vi "Run Action_Do.vi"(8 "error in (no error)":errorcluster, 10 "Project Builder in":refnum<class "Project Builder.lvclass">, 11 "Set Version from Git Tag":refnum<class "Set Version from Git Tag.lvclass">) -> (0 "error out":errorcluster, 1 "Success?":bool, 3 "Report":refnum<class "Report Data.lvclass">)   [LabVIEW 2019, in "ProjectBuilder.lvlib" / "Set Version from Git Tag.lvclass"]
doc: "Run the action associated with the 'Project Action'-class.\n\nThis implementation gets the Git tag and sets the build specification version to the tag version."
uses:
  Set Version from Git Tag.lvclass
  Project Action/Project Action.lvclass
  ProjectBuilder.lvlib
  <vilib>/AppBuilder/AB_API_Simple/Build Specification Version.ctl
  <vilib>/AppBuilder/AB_API_Simple/NI_App_Builder_API.lvlib
  Version Data/Version Data.lvclass
  Data/Report Data/Report Data.lvclass
  Project Builder/Project Builder.lvclass
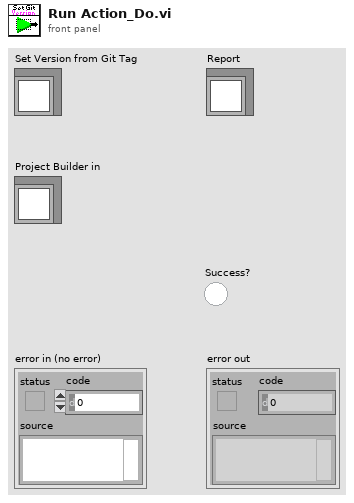
[diagram p1: front panel]
types:
  T1 = typedef "NI_App_Builder_API.lvlib/Build Specification Version.ctl" = cluster{"Major":u16, "Minor":u16, "Fix":u16, "Build":u16}
  T2 = cluster{"Build Specification Version[0]":i32, "Build Specification Version[1]":i32, "Build Specification Version[2]":i32, "Build Specification Version[3]":i32}
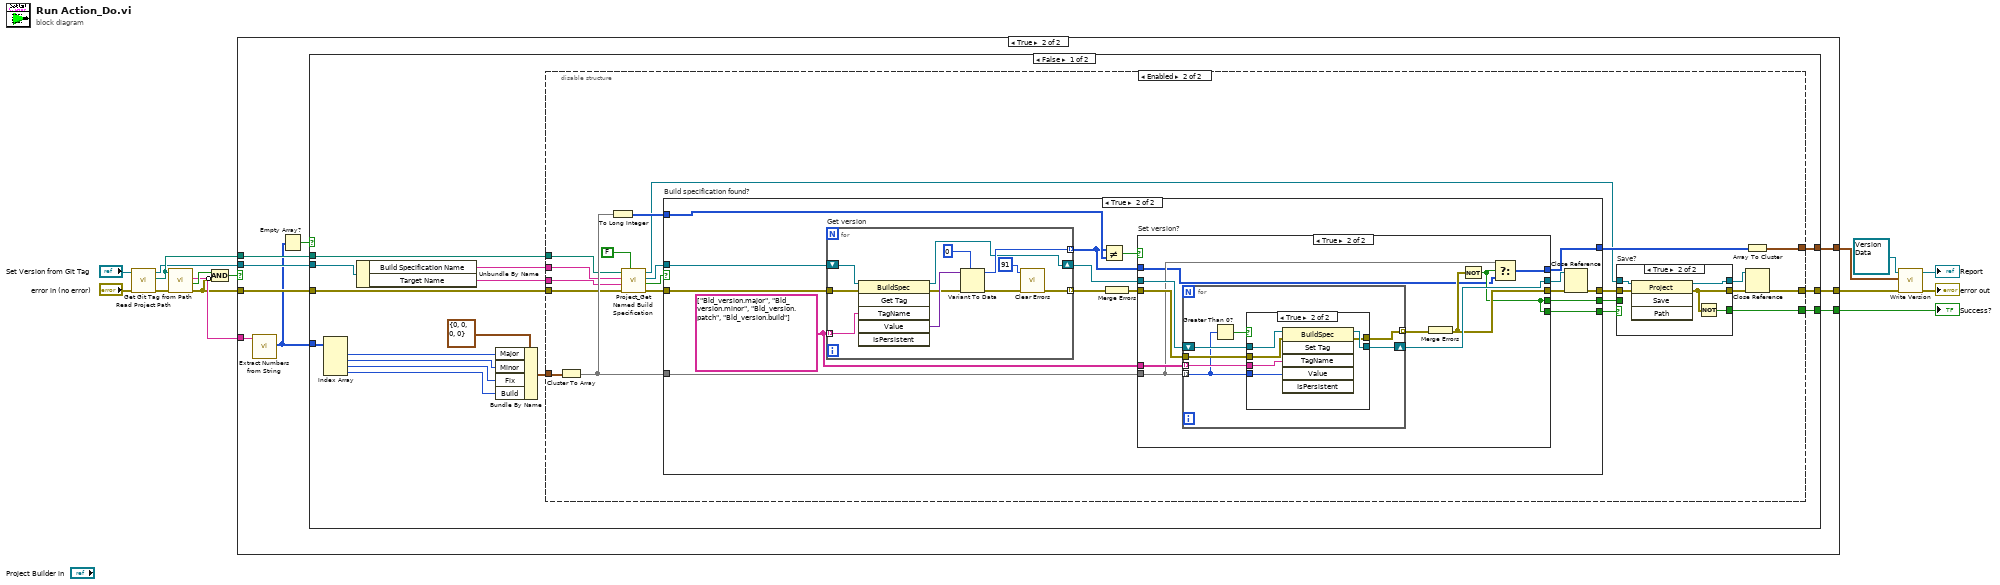
[diagram p0: block diagram]
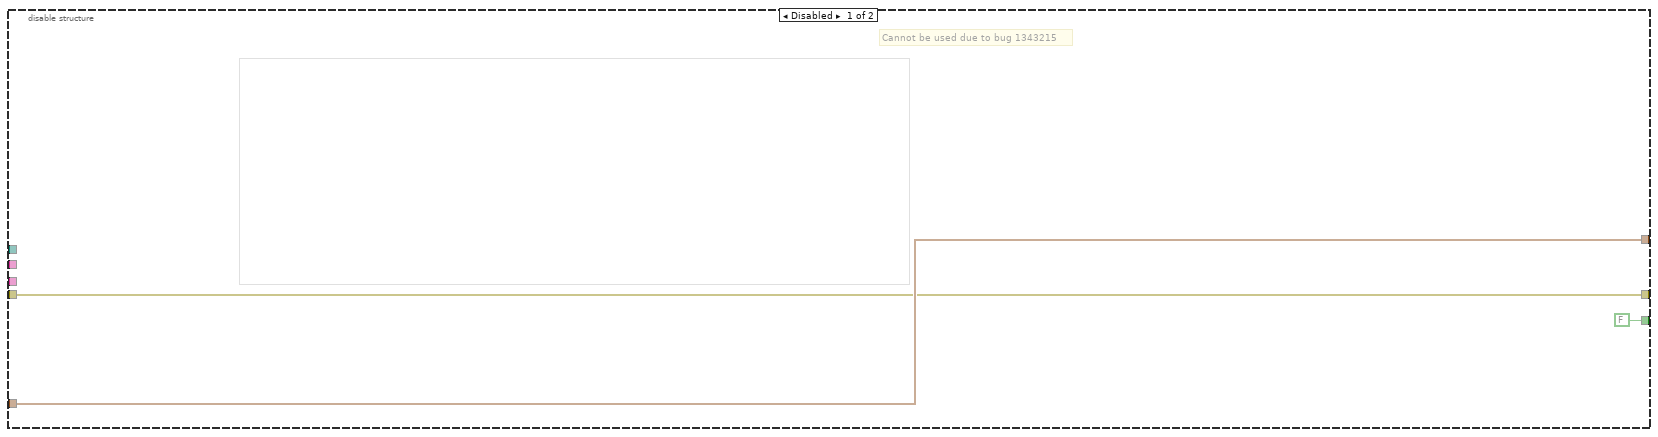
[diagram p3: hidden frame]
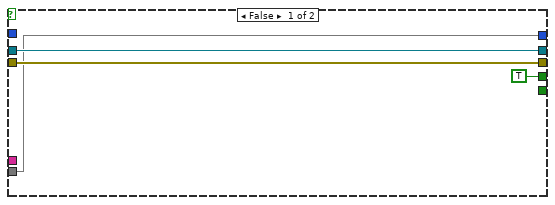
[diagram p5: hidden frame]
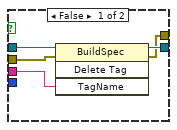
[diagram p6: hidden frame]
diagram:
  n1 = call "Read Project Path.vi"("error in (no error)"="error in (no error)", "Project Action in"="Set Version from Git Tag") -> ("error out"=w13:errorcluster, "Project Path"=w9:path, "Project Action out"=w7:refnum<class "Set Version from Git Tag.lvclass">)  [unwired: 7 in]
  n2 = call "Get Git Tag from Path.vi"("error in (no error)"=w13, "Path"=w9) -> ("error out"=w8:errorcluster, "Success?"=w12:bool, "Tag"=w10:string)  [unwired: 6 in, 1 out]
  n3 = Compound Arithmetic op=AND(w12, invert w8) -> (w11:bool)
  n4 = case shown="True" w11 {
    selector: w11 -> [w16 _]
    tunnel: w10 -> [_ w26]
    tunnel: w9 -> [_ w25]
    tunnel: [w17 w22] -> w6
    tunnel: w8 -> [w17 w23]
    tunnel: [w16 w21] -> w5
    tunnel: w7 -> [_ w24]
    tunnel: [_ w18] -> w1
    frame False {
    }
    frame True {
      n5 = call "Extract Numbers from String.vi"("String"=w26) -> ("Number Array"=w20:i32[])  [unwired: 9 in, 1 out]
      n6 = Empty Array?(array=w20) -> (empty?=w19:bool)
      n7 = case shown="False" w19 {
        tunnel: w25 -> [w28 _]
        tunnel: w24 -> [w36 _]
        tunnel: w23 -> [w29 w134]
        tunnel: [w27 w134] -> w22
        tunnel: [w35 _] -> w21
        tunnel: w20 -> [w34 _]
        tunnel: [w31 _] -> w18
        frame False {
          n8 = Index Array(array=w34) -> (element #1=w40:i32, element #2=w39:i32, element #3=w38:i32, element #4=w37:i32)  [unwired: 4 in]
          n9 = Unbundle By Name(w36) -> ("Build Specification Name"=w33:string, "Target Name"=w30:string)
          n10 = Bundle By Name(cluster=T1 {"Major"=0, "Minor"=0, "Fix"=0, "Build"=0} ("Build Specification Version"), "Major"=w40, "Minor"=w39, "Fix"=w38, "Build"=w37) -> (w32:T1)
          n11 = disable-structure shown="Enabled" {
            disable-tunnel: [FALSE w58] -> w35
            disable-tunnel: w33 -> [_ w53]
            disable-tunnel: w32 -> [w44 w63]
            disable-tunnel: [w44 w55] -> w31
            disable-tunnel: w30 -> [_ w45]
            disable-tunnel: w29 -> [w43 w54]
            disable-tunnel: w28 -> [_ w52]
            disable-tunnel: [w43 w59] -> w27
            frame Disabled {
              # "Cannot be used due to bug 1343215"
            }
            frame Enabled {
              n12 = Cluster To Array(cluster=w63) -> (array=w62:u16[])
              n13 = To Long Integer(number=w62) -> (32bit integer=w61:i32[])
              n14 = call "Project_Get Named Build Specification.vi"("Close project reference(T)"=FALSE, "error in(no error)"=w54, "Target Name(\"\"> My Computer)"=w45, "Build Specification Name"=w53, "Project Path"=w52) -> ("error out"=w48:errorcluster, "Success?"=w50:bool, "Build Spec reference"=w49:refnum<vi>, "Project reference (if not closed)"=w47:refnum<vi>)  [unwired: 3 in]
              n15 = case "Build specification found?" shown="True" w50 {
                tunnel: w48 -> [w66 w67]
                tunnel: [w66 w78] -> w46
                tunnel: w62 -> [_ w75]
                tunnel: w61 -> [_ w73]
                tunnel: [_ w72] -> w60
                tunnel: [_ w71] -> w57
                tunnel: [_ w69] -> w56
                tunnel: w49 -> [_ w68]
                frame False {
                }
                frame True {
                  w76 = string[] ["Bld_version.major", "Bld_version.minor", "Bld_version.patch", "Bld_version.build"]
                  n16 = for "Get version" {
                    tunnel: w76 -> [w124] mode=indexing
                    tunnel: [w121] -> w70 mode=indexing
                    shift-right: [w120] -> w77
                    shift-left: w68 -> [w125]
                    tunnel: [w116] -> w80 mode=indexing
                    tunnel: w67 -> [w117]
                    n17 = invoke class="BuildSpec" method="Get Tag"(reference=w125, error in=w117, "TagName"=w124) -> (reference out=w120:refnum<vi>, error out=w119:errorcluster, "Value"=w123:variant)  [unwired: 3 in, 3 out]
                    n18 = Variant To Data(error in=w119, type=0, Variant=w123) -> (data=w121:i32, error out=w118:errorcluster)
                    n19 = call <vilib>:"Clear Errors.vi"("error in (no error)"=w118, "specific error code to clear (0: all)"=91) -> ("error out"=w116:errorcluster)  [unwired: 4 in, 1 out]
                  }
                  n20 = Not Equal?(x=w70, y=w73) -> (x != y?=w74:bool)
                  n21 = Merge Errors(w80) -> (w81:errorcluster)
                  n22 = case "Set version?" shown="True" w74 {
                    tunnel: [w86 w96] -> w82
                    tunnel: w81 -> [w85 w95]
                    tunnel: [w85 w91] -> w79
                    tunnel: w77 -> [w86 w93]
                    tunnel: w76 -> [_ w92]
                    tunnel: w75 -> [w83 w89]
                    tunnel: [_ w90] -> w72
                    tunnel: [TRUE w90] -> w71
                    tunnel: w70 -> [_ w88]
                    tunnel: [w83 w87] -> w69
                    frame False {
                    }
                    frame True {
                      n23 = for {
                        tunnel: w92 -> [w102] mode=indexing
                        shift-right: [w101] -> w96
                        shift-left: w93 -> [w103]
                        tunnel: w89 -> [w98] mode=indexing
                        tunnel: [w100] -> w94 mode=indexing
                        tunnel: w95 -> [w99]
                        n24 = Greater Than 0?(x=w98) -> (x > 0?=w97:bool)
                        n25 = case shown="True" w97 {
                          tunnel: w103 -> [w108 w114]
                          tunnel: w102 -> [w107 w113]
                          tunnel: [w106 w112] -> w101
                          tunnel: [w104 w111] -> w100
                          tunnel: w99 -> [w105 w110]
                          tunnel: w98 -> [_ w109]
                          frame False {
                            n26 = invoke class="BuildSpec" method="Delete Tag"(reference=w108, error in=w105, "TagName"=w107) -> (reference out=w106:refnum<vi>, error out=w104:errorcluster)  [unwired: 1 in, 2 out]
                          }
                          frame True {
                            n27 = invoke class="BuildSpec" method="Set Tag"(reference=w114, error in=w110, "TagName"=w113, "Value"=w109) -> (reference out=w112:refnum<vi>, error out=w111:errorcluster)  [unwired: 2 in, 4 out]
                          }
                        }
                      }
                      n28 = Merge Errors(w94) -> (w91:errorcluster)
                      n29 = Not(x=w91) -> (.not. x?=w90:bool)
                      n30 = Select(t=w89, s=w90, f=w88) -> (s? t:f=w87:i32[])
                    }
                  }
                  n31 = Close Reference(reference=w82, error in (no error)=w79) -> (error out=w78:errorcluster)
                }
              }
              n32 = case "Save?" shown="True" w60 {
                tunnel: [w127 w129] -> w65
                tunnel: [w128 w133] -> w64
                tunnel: w47 -> [w128 w132]
                tunnel: w46 -> [w127 w131]
                tunnel: [w126 w130] -> w58
                tunnel: w57 -> [w126 _]
                frame False {
                }
                frame True {
                  n33 = invoke class="Project" method="Save"(reference=w132, error in=w131) -> (reference out=w133:refnum<vi>, error out=w129:errorcluster)  [unwired: 2 in, 2 out]
                  n34 = Not(x=w129) -> (.not. x?=w130:bool)
                }
              }
              n35 = Array To Cluster(array=w56) -> (cluster=w55:T2)
              n36 = Close Reference(reference=w64, error in (no error)=w65) -> (error out=w59:errorcluster)
            }
          }
        }
        frame True {
        }
      }
    }
  }
  "Success?" <- w5
  n37 = call "Write Version.vi"("error in (no error)"=w6, "Build Specification Version"=w1, "Version Data in"=refnum<class "Version Data.lvclass"> refnum ("ProjectBuilder.lvlib:Version Data.lvclass")) -> ("error out"=→"error out":errorcluster, "Version Data out"=→"Report":refnum<class "Version Data.lvclass">)  [unwired: 7 in]
